vi "Read OnOff Command.vi"   [LabVIEW 2023, in "Cycler.lvclass"]
uses:
  Cycler.lvclass
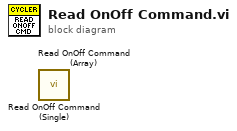
[diagram p0: block diagram]
diagram:
  n1 = call "Read OnOff Command (Single).vi"() -> ()  [unwired: 8 in, 4 out]
  n2 = call "Read OnOff Command (Array).vi"() -> ()  [unwired: 8 in, 4 out]
